vi "SubVI_Process_Gryo.vi"(11 "Bytes Read":u8[](array[numeric])) -> (0 "Temperature (Pure doule precision HW)":dbl, 2 "Gyroscopic Cluster Values":cluster{dbl, dbl, dbl}, 3 "Accelorometer Cluster Values":cluster{i16, i16, i16})   [LabVIEW 2014]
panel:
  out "double precision float":dbl[](array[numeric])
  out "Temp":i16
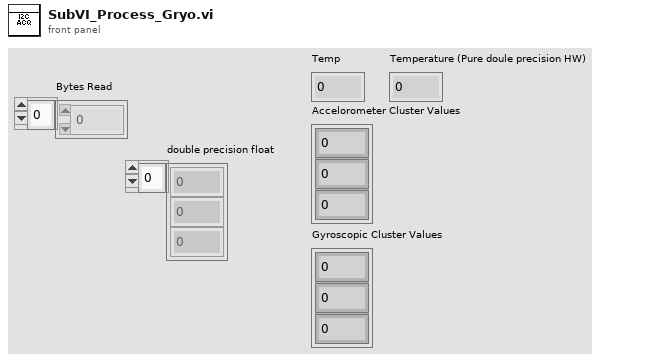
[diagram p1: front panel]
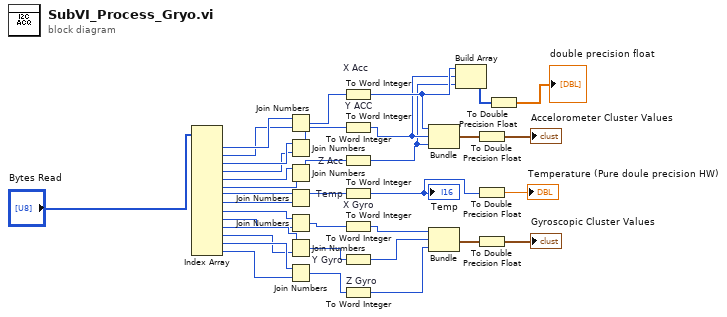
[diagram p0: block diagram]
diagram:
  n1 = Index Array(array="Bytes Read") -> (element #1=w35:u8, element #2=w34:u8, element #3=w33:u8, element #4=w32:u8, element #5=w31:u8, element #6=w30:u8, element #7=w23:u8, element #8=w22:u8, element #9=w24:u8, element #10=w25:u8, element #11=w27:u8, element #12=w26:u8, element #13=w29:u8, element #14=w28:u8)  [unwired: 14 in]
  n2 = Join Numbers(hi=w35, lo=w34) -> ((hi.lo)=w21:u16)
  n3 = Join Numbers(hi=w33, lo=w32) -> ((hi.lo)=w20:u16)
  n4 = Join Numbers(hi=w31, lo=w30) -> ((hi.lo)=w19:u16)
  n5 = Join Numbers(hi=w23, lo=w22) -> ((hi.lo)=w18:u16)
  n6 = Join Numbers(hi=w24, lo=w25) -> ((hi.lo)=w17:u16)
  n7 = Join Numbers(hi=w27, lo=w26) -> ((hi.lo)=w16:u16)
  n8 = Join Numbers(hi=w29, lo=w28) -> ((hi.lo)=w15:u16)
  n9 = To Word Integer "X Acc"(number=w21) -> (16bit integer=w5:i16)
  n10 = To Word Integer "Y ACC"(number=w20) -> (16bit integer=w4:i16)
  n11 = To Word Integer "Z Acc"(number=w19) -> (16bit integer=w3:i16)
  n12 = To Word Integer "Temp"(number=w18) -> (16bit integer=w9:i16)
  "Temp" <- w9
  n13 = To Word Integer "X Gyro"(number=w17) -> (16bit integer=w13:i16)
  n14 = To Word Integer "Y Gyro"(number=w16) -> (16bit integer=w14:i16)
  n15 = To Word Integer "Z Gyro"(number=w15) -> (16bit integer=w12:i16)
  n16 = Bundle(w5, w4, w3) -> (w11:cluster{i16, i16, i16})  [unwired: 1 in]
  n17 = Bundle(w13, w14, w12) -> (w8:cluster{i16, i16, i16})  [unwired: 1 in]
  n18 = Build Array(w5, w4, w3) -> (w2:i16[])
  n19 = To Double Precision Float(number=w11) -> (double precision float=→"Accelorometer Cluster Values":cluster{dbl, dbl, dbl})
  n20 = To Double Precision Float(number=w9) -> (double precision float=→"Temperature (Pure doule precision HW)":dbl)
  n21 = To Double Precision Float(number=w8) -> (double precision float=→"Gyroscopic Cluster Values":cluster{dbl, dbl, dbl})
  n22 = To Double Precision Float(number=w2) -> (double precision float=→"double precision float":dbl[])
